vi "Write error ref.vi"(8 "error in (no error)":errorcluster, 10 "error":refnum<vi>, 11 "GeneralFunctionality in":refnum<class "GeneralFunctionality.lvclass">) -> (0 "error out":errorcluster, 3 "GeneralFunctionality out":refnum<class "GeneralFunctionality.lvclass">)   [LabVIEW 2020, in "GeneralFunctionality.lvclass"]
uses:
  GeneralFunctionality.lvclass
  GeneralFunctionality.lvclass/GeneralFunctionality.ctl
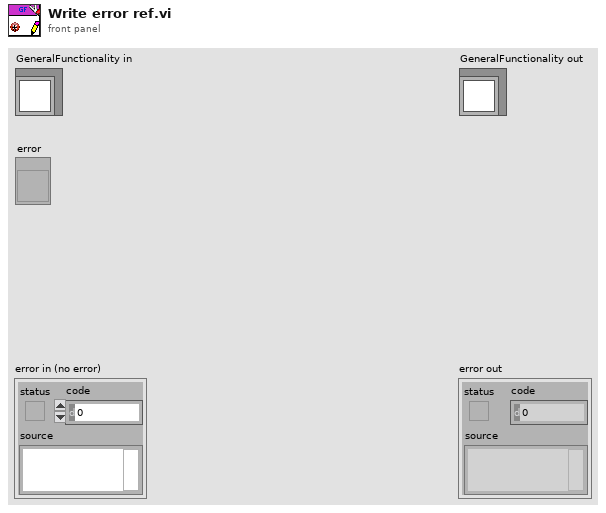
[diagram p1: front panel]
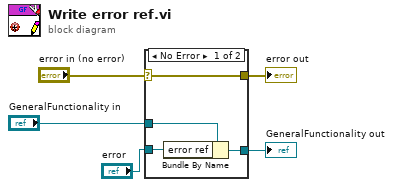
[diagram p0: block diagram]
diagram:
  n1 = case shown="No Error" "error in (no error)" {
    selector: "error in (no error)" -> [w9 w10]
    tunnel: [w9 w10] -> w4
    tunnel: [w7 w11] -> w2
    tunnel: "GeneralFunctionality in" -> [w8 w11]
    tunnel: "error" -> [w6 _]
    frame No Error {
      n2 = Bundle By Name(cluster=w8, "error ref"=w6) -> (w7:refnum<class "GeneralFunctionality.lvclass">)
    }
    frame Error {
    }
  }
  "error out" <- w4
  "GeneralFunctionality out" <- w2
